vi "Async.Engine.DynamicConfigInitialize.vi"(8 "error in":errorcluster, 10 "Data Access info":T3 {"Read"."Refs"."Data Reference" format="%.0x"; "Write"."Refs"."Data Reference" format="%.0x"; "ReadWrite"."Refs" format="%.0x"}, 11 "Async in":refnum<class "VS Inline Async API.lvclass">) -> (0 "error out":errorcluster, 3 "Async out":refnum<class "VS Inline Async API.lvclass">)   [LabVIEW 2023, in "VS Inline Async API.lvlib" / "VS Inline Async API.lvclass"]
uses:
  VS Inline Async API.lvclass
  VS Inline Async API.lvclass/VS Inline Async API.ctl
  _Data Access Engine/Data Access Engine/Data Access Engine.lvclass
  <vilib>/NI VeriStand/Custom Device API/Data Reference.ctl
  <vilib>/NI VeriStand/Custom Device API/Custom Device API.lvlib
  <vilib>/NI VeriStand/Custom Device API/Block Data Reference.ctl
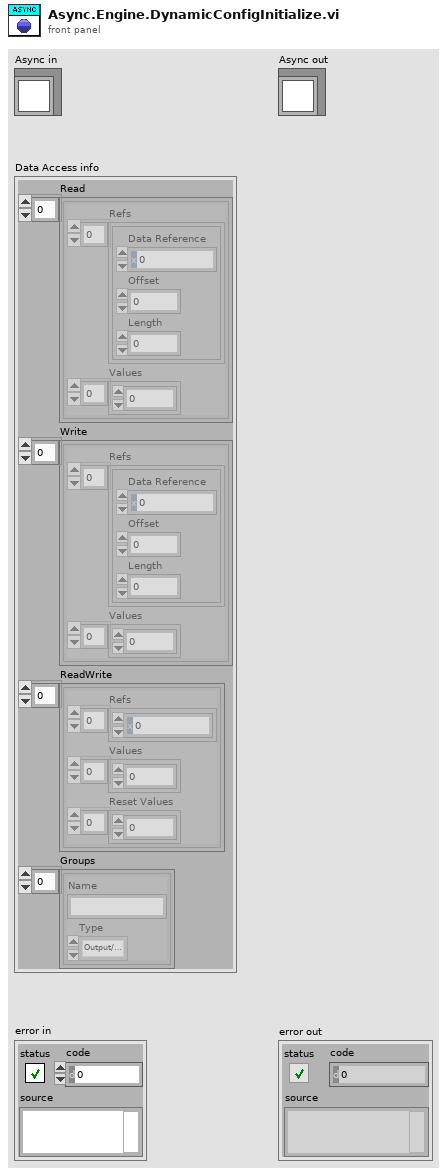
[diagram p1: front panel]
types:
  T1 = typedef "Custom Device API.lvlib/Block Data Reference.ctl" = cluster{"Data Reference":T2, "Offset":u64, "Length":u64}
  T2 = typedef "Custom Device API.lvlib/Data Reference.ctl" = i32
  T3 = cluster{"Read":cluster{"Refs":T1[], "Values":dbl[]}[], "Write":cluster{"Refs":T1[], "Values":dbl[]}[], "ReadWrite":cluster{"Refs":T2[], "Values":dbl[], "Reset Values":dbl[]}[], "Groups":cluster{"Name":string, "Type":enum16{"Output/Write", "Input/Read", "Input/ReadWrite"}}[]}
  T4 = enum16{"Initialize", "Start", "Read Data from hardware", "Write Data to hardware", "Close", "Get State"}
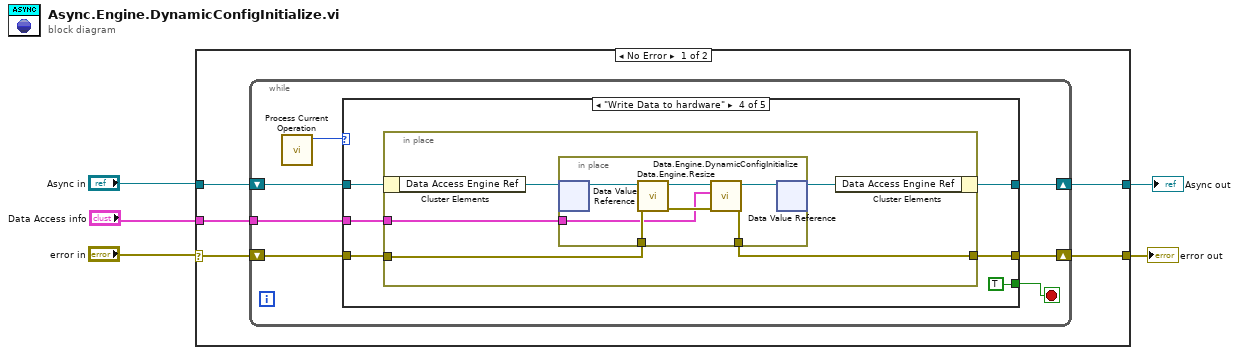
[diagram p0: block diagram]
diagram:
  n1 = case shown="No Error" "error in" {
    selector: "error in" -> [w9 w45]
    tunnel: "Async in" -> [w6 w44]
    tunnel: [w10 w45] -> w4
    tunnel: "Data Access info" -> [w8 _]
    tunnel: [w7 w44] -> w1
    frame No Error {
      n2 = while {
        tunnel: w8 -> [w15]
        shift-right: [w17] -> w10
        shift-left: w9 -> [w16]
        shift-right: [w14] -> w7
        shift-left: w6 -> [w13]
        stop <- w12 stop-if-true
        n3 = call "Process Current Operation.vi"() -> ("Current Operation out"=w11:T4)  [unwired: 10 in, 1 out]
        n4 = case shown="\"Write Data to hardware\"" w11 {
          tunnel: [w19 w21 w23 w29 w43] -> w17
          tunnel: w15 -> [_ _ _ w27 _]
          tunnel: w16 -> [w19 w21 w23 w28 w43]
          tunnel: [w18 w20 w22 w26 w42] -> w14
          tunnel: w13 -> [w18 w20 w22 w25 w42]
          tunnel: [_ _ _ TRUE _] -> w12
          frame "Initialize", Default {
          }
          frame "Start" {
          }
          frame "Read Data from hardware" {
          }
          frame "Write Data to hardware" {
            n5 = in-place {
              in-place-border: w28 -> [w33]
              in-place-border: [w34] -> w29
              in-place-border: w27 -> [w32]
              n6 = in-place-cluster #1(w25) -> ("Data Access Engine Ref"=w31:refnum<data-value>)
              n7 = in-place {
                in-place-border: [w41] -> w34
                in-place-border: w32 -> [w38]
                in-place-border: w33 -> [w39]
                n8 = in-place-dvr #2(w31) -> (w36:refnum<class "Data Access Engine.lvclass">)  [unwired: 1 out]
                n9 = call "Data.Engine.Resize.vi"("error in"=w39, "Data Access API in"=w36) -> ("error out"=w40:errorcluster, "Data Access API out"=w35:refnum<class "Data Access Engine.lvclass">)  [unwired: 8 in]
                n10 = call "Data.Engine.DynamicConfigInitialize.vi"("error in"=w40, "Data Access info"=w38, "Data Access Engine"=w35) -> ("error out"=w41:errorcluster, "Data Access Engine"=w37:refnum<class "Data Access Engine.lvclass">)  [unwired: 7 in]
                n11 = in-place-dvr #2(w37) -> (w30:refnum<data-value>)  [unwired: 1 out]
              }
              n12 = in-place-cluster #1("Data Access Engine Ref"=w30) -> (w26:refnum<class "VS Inline Async API.lvclass">)
            }
          }
          frame "Close" {
          }
        }
      }
    }
    frame Error {
    }
  }
  "error out" <- w4
  "Async out" <- w1
